vi "Stop HTTP.vi"(8 "error in (no error)":errorcluster, 11 "Vecto in":refnum<class "Vecto.lvclass">) -> (0 "error out":errorcluster, 3 "Vecto out":refnum<class "Vecto.lvclass">)   [LabVIEW 2020, in "Vecto.lvlib" / "Vecto.lvclass"]
uses:
  Vecto.lvclass
  proto/ServiceType/Enumeration.ctl
  Vecto.lvclass/Vecto.ctl
  <vilib>/IlluminatedG/IG HTTP Server/HTTP Server/Server/Server.lvclass
  VectoService/VectoService.lvclass
  DiscoveryService/DiscoveryService.lvclass
  proto/ServiceType/ServiceType.lvlib
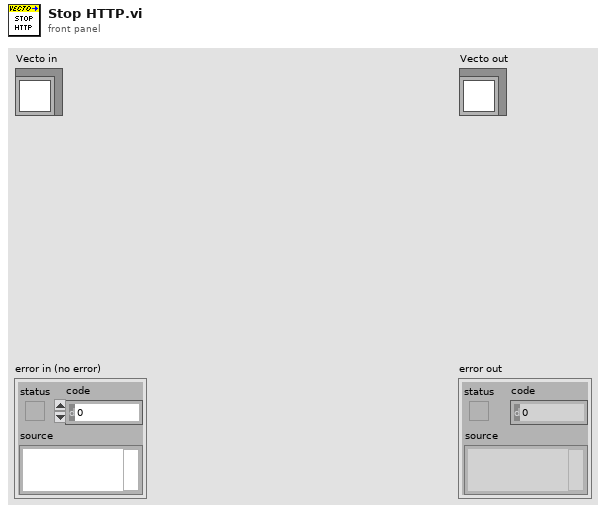
[diagram p1: front panel]
types:
  T1 = typedef "ServiceType.lvlib/Enumeration.ctl" = enum16{"SERVICETYPE_UNKNOWN", "SERVICETYPE_TCPSERVER", "SERVICETYPE_HTTPSERVER"}
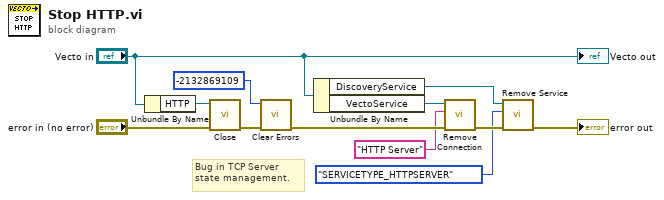
[diagram p0: block diagram]
diagram:
  # "Bug in TCP Server state management."
  n1 = Unbundle By Name("Vecto in") -> ("HTTP"=w11:refnum<class "Server.lvclass">)
  n2 = call <vilib>:"Close.vi"("error in (no error)"="error in (no error)", "Server in"=w11) -> ("error out"=w9:errorcluster)  [unwired: 8 in, 1 out]
  n3 = call <vilib>:"Clear Errors.vi"("error in (no error)"=w9, "specific error code to clear (0: all)"=-2132869109) -> ("error out"=w12:errorcluster)  [unwired: 4 in, 1 out]
  n4 = Unbundle By Name("Vecto in") -> ("DiscoveryService"=w3:refnum<class "DiscoveryService.lvclass">, "VectoService"=w6:refnum<class "VectoService.lvclass">)
  n5 = call "Remove Connection.vi"("error in (no error)"=w12, "Connection Name"="HTTP Server", "VectoService in"=w6) -> ("error out"=w5:errorcluster)  [unwired: 7 in, 1 out]
  n6 = call "Remove Service.vi"("error in (no error)"=w5, "Service Type"=Enumeration."SERVICETYPE_HTTPSERVER", "DiscoveryService in"=w3) -> ("error out"=→"error out":errorcluster)  [unwired: 7 in, 1 out]
  "Vecto out" <- "Vecto in"
